vi "MainPC.vi"() -> ()   [LabVIEW 2017]
doc: "Use this template to build a simple state machine design pattern. Each state executes code and determines which state to transition to."
uses:
  Projekt-RubikLibrary/SingmasterAllMoves.ctl
  TypeDefs/UIState.ctl
  TypeDefs/CommandsRT.ctl
  Projekt-RubikLibrary/RubikLibrary.lvlib
panel:
  in  "Singmaster Move":T1=enum."L"
  in  "Rotate Button":bool
  in  "Exit":bool
  # "Rubik's Cube Orientation"
  # "Rotates Cube around \nLeft-Right axis.\n\nRun MainRT on myRIO!"
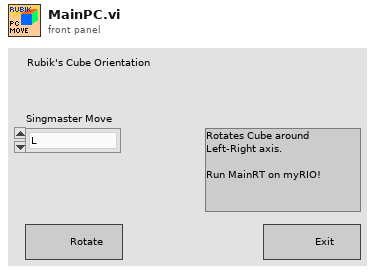
[diagram p1: front panel]
types:
  T1 = typedef "RubikLibrary.lvlib/SingmasterAllMoves.ctl" = enum16{"U", "L", "F", "R", "B", "D", "U'", "L'", "F'", "R'", "B'", "D'"}
  T2 = typedef "UIState.ctl" = enum16{"Initializing", "Wait for Event", "Rotating", "Exiting"}
  T3 = typedef "CommandsRT.ctl" = enum16{"Initialize", "Rotate", "Exit"}
  T4 = typedef "DataStreamCluster.ctl" = cluster{"Commands":T3, "Variant":variant}
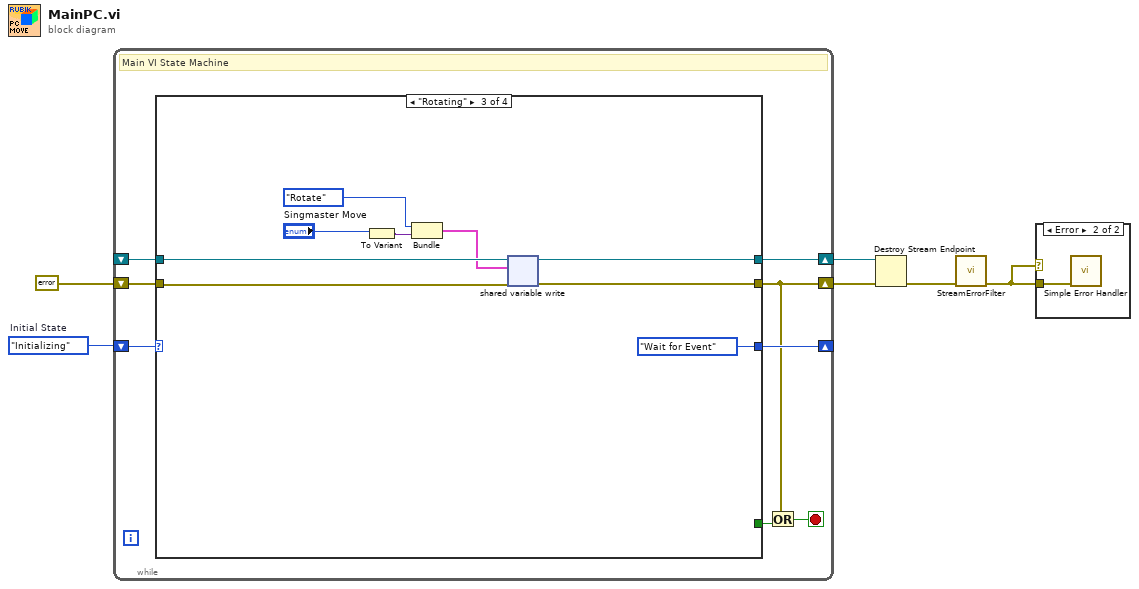
[diagram p0: block diagram]
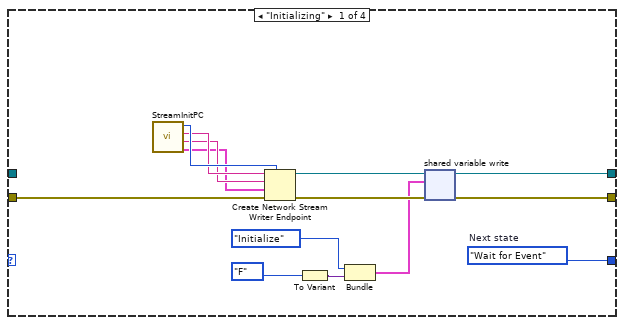
[diagram p3: hidden frame]
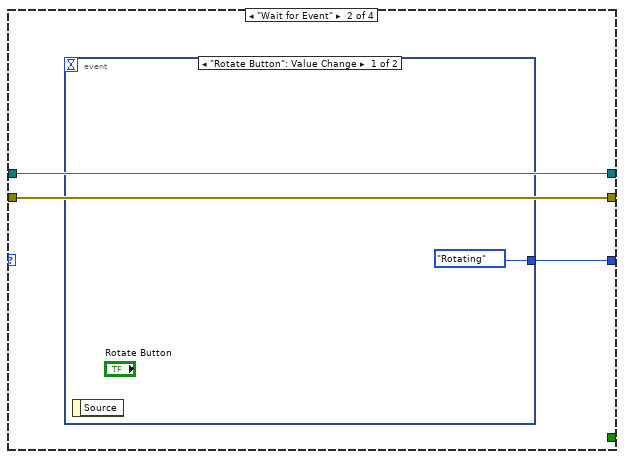
[diagram p4: hidden frame]
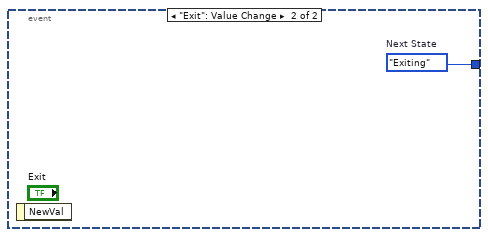
[diagram p5: hidden frame]
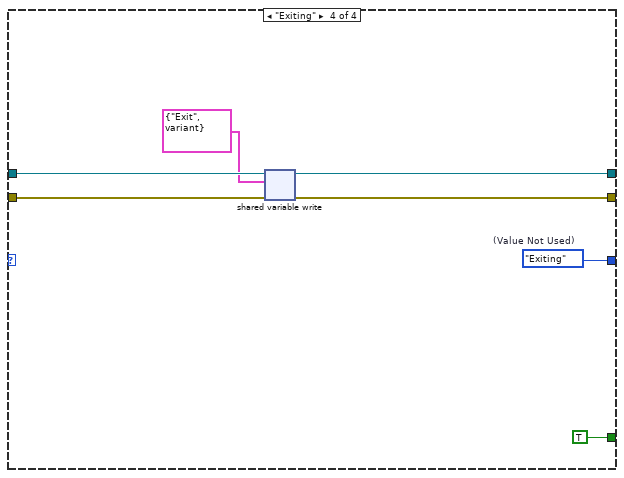
[diagram p6: hidden frame]
diagram:
  w6 = UIState."Initializing"  # Initial State
  n1 = while {
    shift-right: [w14] -> _
    shift-left: w6 -> [w11]
    shift-right: [w7] -> w4
    shift-left: errorcluster {"status"=FALSE, "code"=0, "source"=""} ("error constant") -> [w10]
    shift-right: [w9] -> w3
    shift-left: _ -> [w8]
    stop <- w12 stop-if-true
    # "Main VI State Machine"
    n2 = case shown="\"Rotating\"" w11 {
      tunnel: [w28 w31 UIState."Wait for Event" ("(Value Not Used)") w49] -> w14
      tunnel: [_ _ _ TRUE ("Stop Loop?")] -> w13
      tunnel: [w19 w29 w40 w46] -> w7
      tunnel: w10 -> [w24 w29 w41 w47]
      tunnel: [w17 w30 w39 w45] -> w9
      tunnel: w8 -> [_ w30 w38 w44]
      frame "Initializing" {
        w28 = UIState."Wait for Event"  # Next state
        # "Initialize - Initialize the application."
        n3 = call "StreamInitPC.vi"() -> ("data cluster"=w23:T4, "reader name"=w25:string, "writer name"=w26:string, "writer buffer size"=w27:i32)  [unwired: 4 in]
        n4 = Create Network Stream Writer Endpoint(7:w27, 8:w24, 9:w23, 10:w25, 11:w26) -> (0:w20:errorcluster, 3:w18:refnum<k21>)  [unwired: 2 in]
        n5 = To Variant(anything=SingmasterAllMoves."F" ("Singmaster Move 2")) -> (Variant=w21:variant)
        n6 = Bundle("Commands"=CommandsRT."Initialize", "Variant"=w21) -> (w16:cluster{"Commands":T3, "Variant":variant})  [unwired: 1 in]
        n7 = shared-variable-write(w18, w20, w16) -> (w17:refnum<k21>, w19:errorcluster)  [unwired: 1 in, 1 out]
      }
      frame "Wait for Event" {
        # "Wait for Event - Use an Event Structure to monitor the user interface for events that run different states of the state machine."
        n8 = event shown="[0] \"Rotate Button\": Value Change" {
          selector: _ -> [_ _]
          dyn-events: _ -> [_ _]
          timeout: _ -> [_ _]
          tunnel: [UIState."Rotating" ("Next State") w33] -> w31
          event "Rotate Button": Value Change {
            n9 = event-data() -> ()  [unwired: 1 in, 1 out]
          }
          event "Exit": Value Change {
            w33 = UIState."Exiting"  # Next State
            n10 = event-data() -> ()  [unwired: 1 in, 1 out]
          }
        }
      }
      frame "Rotating" {
        n11 = To Variant(anything="Singmaster Move") -> (Variant=w36:variant)
        n12 = Bundle("Commands"=CommandsRT."Rotate", "Variant"=w36) -> (w35:cluster{"Commands":T3, "Variant":variant})  [unwired: 1 in]
        n13 = shared-variable-write(w38, w41, w35) -> (w39:refnum<k21>, w40:errorcluster)  [unwired: 1 in, 1 out]
      }
      frame "Exiting" {
        w49 = UIState."Exiting"  # (Value Not Used)
        n14 = shared-variable-write(w44, w47, cluster{"Commands":T3, variant} {"Commands"=enum."Exit", variant} ("anything")) -> (w45:refnum<k21>, w46:errorcluster)  [unwired: 1 in, 1 out]
      }
    }
    n15 = Or(x=w7, y=w13) -> (x .or. y?=w12:bool)
  }
  n16 = Destroy Stream Endpoint(8:w4, 11:w3) -> (0:w5:errorcluster)
  n17 = call "StreamErrorFilter.vi"("error in (no error)"=w5) -> ("error out"=w1:errorcluster)  [unwired: 10 in]
  n18 = case shown="Error" w1 {
    tunnel: w1 -> [_ w50]
    frame No Error {
    }
    frame Error {
      n19 = call <vilib>:"Simple Error Handler.vi"("error in (no error)"=w50) -> ()  [unwired: 4 in, 5 out]
    }
  }
